vi "Update Event Queue Nested.vi"(9 "Insert (T) or Remove (F)":bool, 10 "Queue Nested":map{string, refnum<data-value>}(c390), 11 "Base Queue Actor in":refnum<class "Base Queue Actor.lvclass">) -> (3 "Base Queue Actor out":refnum<class "Base Queue Actor.lvclass">)   [LabVIEW 2021, in "jettl.lvlib" / "Base Queue Actor.lvclass"]
uses:
  Base Queue Actor.lvclass
  Msg/Msg/Msg.lvclass
  Msg/Msgs/Update Queue Nested/Update Queue Nested Msg/Update Queue Nested Msg.lvclass
  C:/git/jettl/src/jettl/Msg/Msg.lvclass
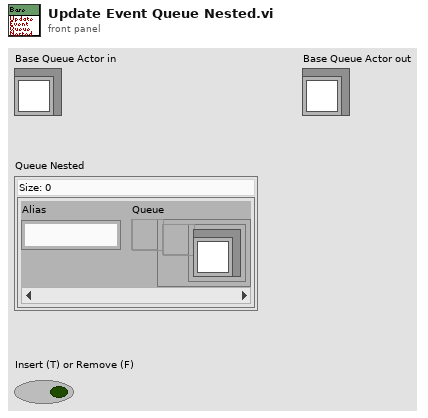
[diagram p1: front panel]
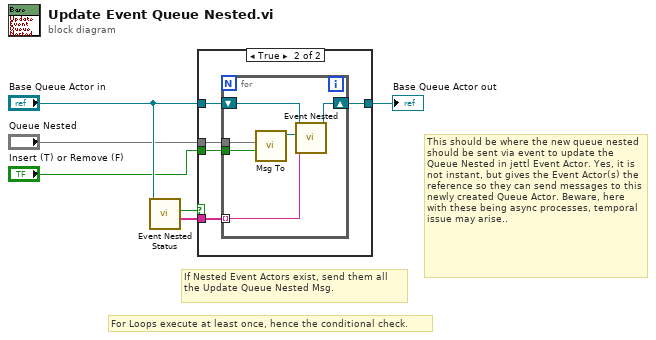
[diagram p0: block diagram]
diagram:
  # "This should be where the new queue nested should be sent via event to update the Queue Nested in jettl Event Actor. Yes, it is not instant, but gives the Event Actor(s) the reference so they can send messages to this newly created Queue Actor. Beware, here with these being async processes, temporal issue may arise.."
  # "If Nested Event Actors exist, send them all the Update Queue Nested Msg."
  # "For Loops execute at least once, hence the conditional check."
  n1 = call-dynamic "Event Nested Status.vi"("Base Queue Actor in"="Base Queue Actor in") -> ("Event Nested Aliases"=w5:string[], "Any Exist?"=w6:bool)  [unwired: 8 in, 1 out]
  n2 = case shown="True" w6 {
    tunnel: [w7 w12] -> w3
    tunnel: "Base Queue Actor in" -> [w7 w11]
    tunnel: w5 -> [_ w10]
    tunnel: "Queue Nested" -> [_ w9]
    tunnel: "Insert (T) or Remove (F)" -> [_ w8]
    frame False {
    }
    frame True {
      n3 = for {
        tunnel: w10 -> [w16] mode=indexing
        shift-right: [w17] -> w12
        shift-left: w11 -> [w18]
        tunnel: w9 -> [w15]
        tunnel: w8 -> [w13]
        n4 = call "Msg To.vi"("Insert (T) or Remove (F)"=w13, "Queue Nested"=w15) -> ("Update Queue Nested Msg out"=w14:refnum<class "Update Queue Nested Msg.lvclass">)  [unwired: 9 in]
        n5 = call-dynamic "Event Nested.vi"("Alias"=w16, "Msg"=w14, "Base Queue Actor in"=w18) -> ("Base Queue Actor out"=w17:refnum<class "Base Queue Actor.lvclass">)  [unwired: 8 in]
      }
    }
  }
  "Base Queue Actor out" <- w3
